vi "Add Client Certificate Paths.vi"(10 "Client Connection Configuration In":T1) -> (2 "Client Connection Configuration Out":T1)   [LabVIEW 2013, in "OPC UA Client Tests.lvlib"]
doc: "Add Certificate paths to Client configuration"
uses:
  OPC UA Client Tests.lvlib
  module/configuration/Client Connection Configuration.ctl
  module/configuration/OPC UA Client configuration.lvclass
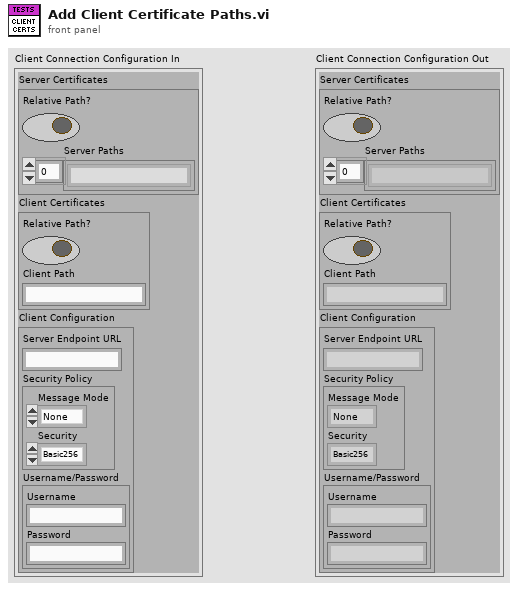
[diagram p1: front panel]
types:
  T1 = typedef "OPC UA Client configuration.lvclass/Client Connection Configuration.ctl" = cluster{"Server Certificates":cluster{"Relative Path?":bool, "Server Paths":string[]}, "Client Certificates":cluster{"Relative Path?":bool, "Client Path":string}, "Client Configuration":cluster{"Server Endpoint URL":string, "Security Policy":cluster{"Message Mode":enum16{"None", "Sign", "Sign and Encrypt"}, "Security":enum16{"Basic256", "Basic128Rsa15"}}, "Username/Password":cluster{"Username":string, "Password":string}}}
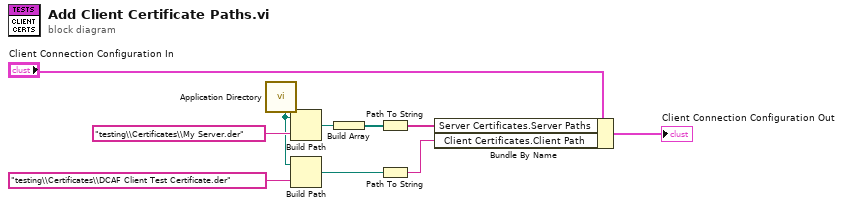
[diagram p0: block diagram]
diagram:
  n1 = call <vilib>:"Application Directory.vi"() -> ("Application Directory"=w6:path)
  n2 = Build Path(base path=w6, name or relative path="testing\\Certificates\\My Server.der") -> (appended path=w9:path)
  n3 = Build Path(base path=w6, name or relative path="testing\\Certificates\\DCAF Client Test Certificate.der") -> (appended path=w1:path)
  n4 = Build Array(w9) -> (w10:path[])
  n5 = Path To String(path=w10) -> (string=w3:string[])
  n6 = Path To String(path=w1) -> (string=w2:string)
  n7 = Bundle By Name(cluster="Client Connection Configuration In", "Server Certificates.Server Paths"=w3, "Client Certificates.Client Path"=w2) -> (→"Client Connection Configuration Out":T1)
